vi "Get UI Details.vi"(8 "error in":errorcluster) -> (0 "error out":errorcluster, 3 "UserInterfaceDetails":T1)   [LabVIEW 2020, in "Line Regulation.lvlib"]
uses:
  Line Regulation.lvlib
  RPC Messages/ni_measurements_v1_UserInterfaceDetails.ctl
  Measurement UI.vi
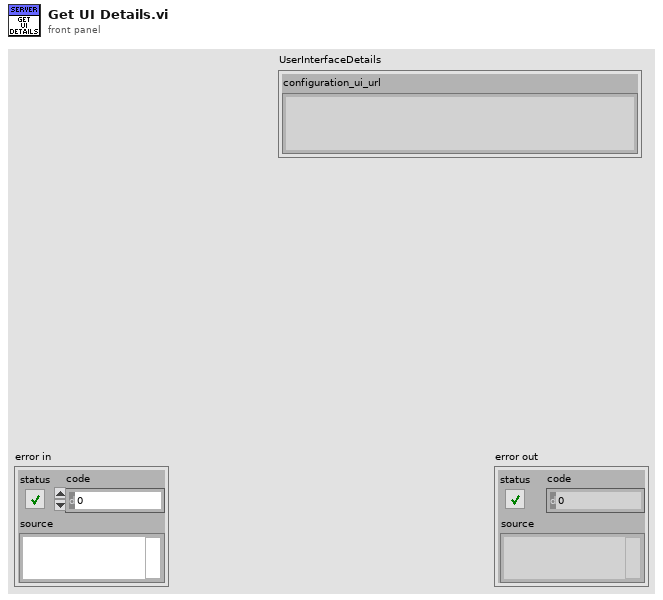
[diagram p1: front panel]
types:
  T1 = typedef "Line Regulation.lvlib/ni_measurements_v1_UserInterfaceDetails.ctl" = cluster{"configuration_ui_url":string}
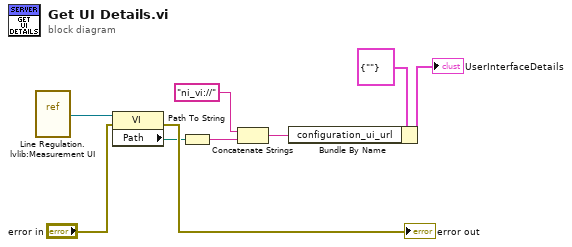
[diagram p0: block diagram]
diagram:
  n1 = vi-ref "Line Regulation.lvlib:Measurement UI.vi"() -> (w9:refnum<vi>)
  n2 = property class="VI"(reference=w9, error in="error in") -> (error out=→"error out":errorcluster, "Path"=w6:path)  [unwired: 1 out]
  n3 = Path To String(path=w6) -> (string=w3:string)
  n4 = Concatenate Strings("ni_vi://" ("string"), w3) -> (w2:string)
  n5 = Bundle By Name(cluster=T1 {"configuration_ui_url"=""} ("UserInterfaceDetails"), "configuration_ui_url"=w2) -> (→"UserInterfaceDetails":T1)
